vi "dfd_Sort Array based on Real Part.vi"(11 "input array":cdb[](array[numeric])) -> (2 "start negtive index":i32, 3 "sorted array":cdb[](array[numeric]))   [LabVIEW 2017, in "NI_DigFilter_Design.lvlib"]
uses:
  <vilib>/addons/Digital Filter Design/NI_DigFilter_Design.lvlib
panel:
  out "set":bool
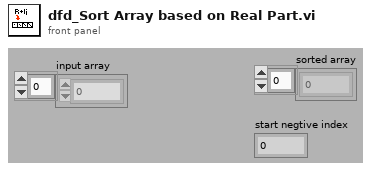
[diagram p1: front panel]
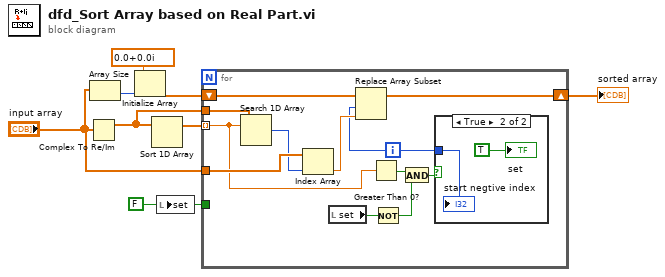
[diagram p0: block diagram]
diagram:
  w3 = FALSE ("set")
  n1 = Complex To Re/Im(x + iy="input array") -> (x=w5:dbl[])  [unwired: 1 out]
  n2 = Array Size(array="input array") -> (size(s)=w7:i32)
  n3 = Initialize Array(cdb 0.0+0.0i, w7) -> (w6:cdb[])
  n4 = Sort 1D Array(array=w5) -> (sorted array=w4:dbl[])
  n5 = local write "set"(w3) -> ()
  n6 = for {
    tunnel: "input array" -> [w20]
    shift-right: [w17] -> w2
    shift-left: w6 -> [w18]
    tunnel: w5 -> [w16]
    tunnel: w4 -> [w14] mode=indexing
    tunnel: w3 -> [_]
    i -> [w13]
    n7 = Search 1D Array(1D array=w16, element=w14) -> (index of element=w19:i32)  [unwired: 1 out]
    n8 = Index Array(array=w20, index=w19) -> (element=w15:cdb)
    n9 = local read "set"() -> (w11:bool)
    n10 = Replace Array Subset(array=w18, new element=w15, index=w13) -> (w17:cdb[])
    n11 = Greater Than 0?(x=w14) -> (x > 0?=w12:bool)
    n12 = Not(x=w11) -> (.not. x?=w9:bool)
    n13 = And(x=w12, y=w9) -> (x .and. y?=w10:bool)
    n14 = case shown="True" w10 {
      tunnel: w13 -> [_ w21]
      frame False {
      }
      frame True {
        "set" <- TRUE ("set")
        "start negtive index" <- w21
      }
    }
  }
  "sorted array" <- w2
